vi "Verify Calibration.vi"(8 "error in":errorcluster, 11 "Instruments in":refnum<class "Instruments.lvclass">) -> (0 "error out":errorcluster, 3 "Instruments out":refnum<class "Instruments.lvclass">)   [LabVIEW 2023, in "Instruments.lvlib" / "Instruments.lvclass"]
doc: "This routine will generate a warning when an instrument is due for calibration;\nIt will also generate a warning if an instrument is out of its calibration cycle entirely.\n\nNo errors will be thrown since there is an opportunity to test with instruments out of calibration."
uses:
  Library/Instruments.lvclass
  C:/Users/Public/Documents/Development/builds/Framework/Actor Framework.lvlibp/1abvi3w/vi.lib/ActorFramework/Actor/Actor.lvclass
  Library/Instruments.lvclass/Instruments.ctl
  builds/Framework/Actor Framework.lvlibp/1abvi3w/vi.lib/ActorFramework/Actor/Read Actor Label.vi
  <vilib>/Utility/error.llb/Error Cluster From Error Code.vi
  <vilib>/ErrorRing/Error Ring.xnode
  builds/Framework/Engine.lvlibp/Engine/Library/Engine.lvclass
  C:/Users/Public/Documents/Development/builds/Framework/Engine.lvlibp/Engine/Library/Engine.lvclass
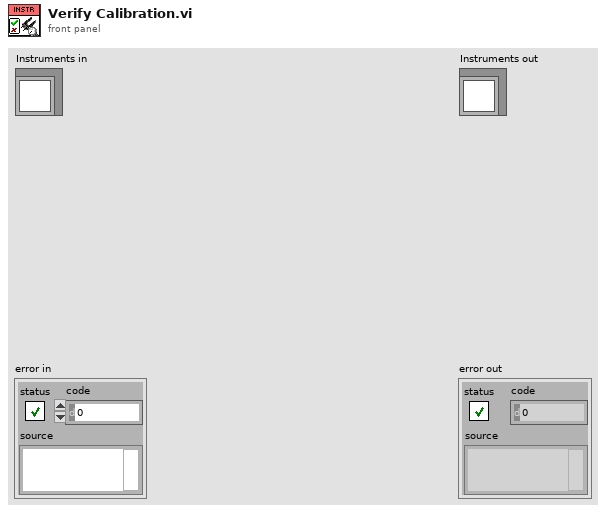
[diagram p1: front panel]
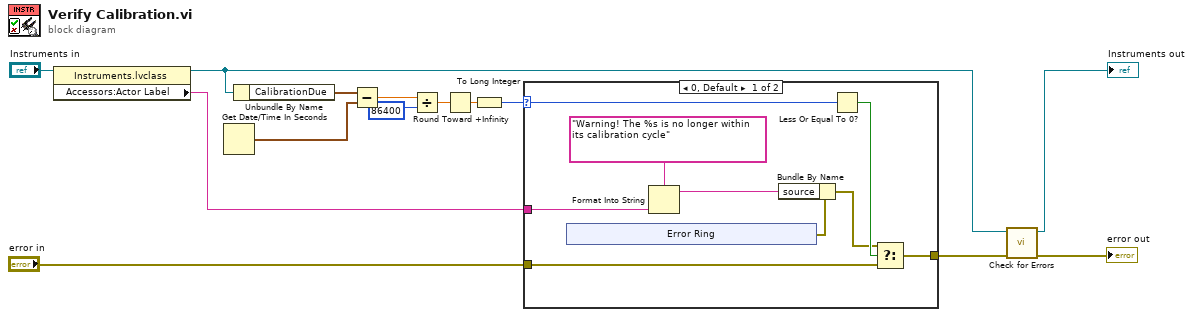
[diagram p0: block diagram]
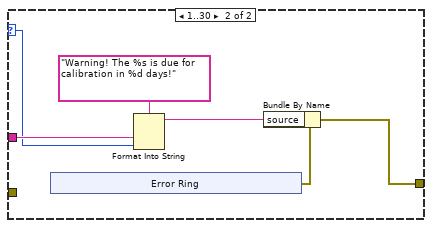
[diagram p2: hidden frame]
diagram:
  n1 = property class="Instruments.lvclass"(reference="Instruments in") -> (reference out=w1:refnum<class "Instruments.lvclass">, "Accessors:Actor Label"=w6:string)  [unwired: 1 in, 1 out]
  n2 = Get Date/Time In Seconds() -> (seconds since 1Jan1904=w11:timestamp)
  n3 = Unbundle By Name(w1) -> ("CalibrationDue"=w4:timestamp)
  n4 = Subtract(x=w4, y=w11) -> (x-y=w14:dbl)
  n5 = Divide(x=w14, y=86400) -> (x/y=w13:dbl)
  n6 = Round Toward +Infinity(x=w13) -> (ceil(x): smallest int >= x=w9:dbl)
  n7 = To Long Integer(number=w9) -> (32bit integer=w12:i32)
  n8 = case shown="0, Default" w12 {
    selector: w12 -> [w19 w28]
    tunnel: "error in" -> [w16 _]
    tunnel: [w15 w32] -> w5
    tunnel: w6 -> [w22 w31]
    frame 0, Default {
      n9 = xnode "Error Ring"() -> ("error out"=w23:errorcluster)
      n10 = Format Into String(format string="Warning! The %s is no longer within its calibration cycle", w22) -> (resulting string=w21:string)  [unwired: 2 in, 1 out]
      n11 = Bundle By Name(cluster=w23, "source"=w21) -> (w17:errorcluster)
      n12 = Less Or Equal To 0?(x=w19) -> (x <= 0?=w18:bool)
      n13 = Select(t=w17, s=w18, f=w16) -> (s? t:f=w15:errorcluster)
    }
    frame 1..30 {
      n14 = xnode "Error Ring"() -> ("error out"=w33:errorcluster)
      n15 = Format Into String(format string="Warning! The %s is due for calibration in %d days!", w31, w28) -> (resulting string=w30:string)  [unwired: 2 in, 1 out]
      n16 = Bundle By Name(cluster=w33, "source"=w30) -> (w32:errorcluster)
    }
  }
  n17 = call "Check for Errors.vi"("error in"=w5, "Engine in"=w1) -> ("error out"=→"error out":errorcluster, "Engine out"=→"Instruments out":refnum<class "Instruments.lvclass">)  [unwired: 8 in]
